vi "example_send_receive_raw.vi"() -> ()   [LabVIEW 2012]
doc: "EXAMPLE: Send / Receive Raw Data\n\nThis example VI allows the user to send and receive raw commands as outlined in the ASCII Language Specification of the USB Communication documentation. Simply key in the \"raw\" command string in the \"command (raw)\" field and run the VI to see the response.\n\nProduced By:\n\nChristopher Lemieux\nKod Integrations, LLC\n4835 Marianne Drive\nMount Airy, MD 21771\nhttp://www.kodintegrations.com\nemail: clemieux@kodintegrations.com\nphone: (240) 687-1288"
panel:
  in  "command (raw)":string
  in  "device_index (def=0)":i32
  out "response (raw)":string
  out "error out":errorcluster
  in  "error in (no error)":errorcluster
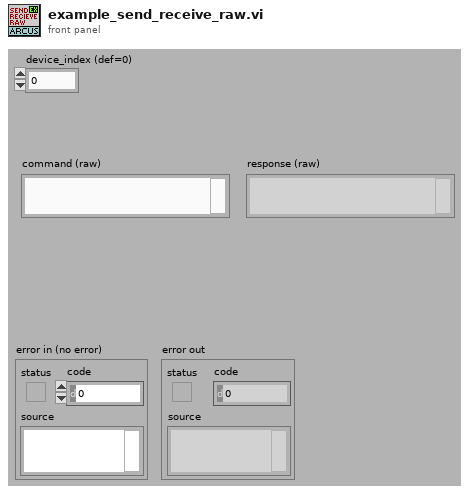
[diagram p1: front panel]
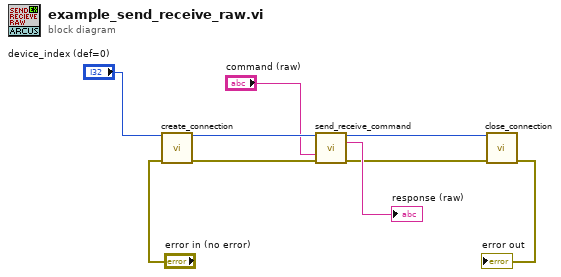
[diagram p0: block diagram]
diagram:
  n1 = call "create_connection.vi"("device_index (def=0)"="device_index (def=0)", "error in (no error)"="error in (no error)") -> ("reference"=w9:i32, "error out"=w8:errorcluster)  [unwired: 12 in]
  n2 = call "send_receive_command.vi"("reference (in)"=w9, "command (raw)"="command (raw)", "error in (no error)"=w8) -> ("reference (dup)"=w2:i32, "read_string"=→"response (raw)":string, "error out"=w3:errorcluster)  [unwired: 8 in, 2 out]
  n3 = call "close_connection.vi"("reference"=w2, "error in (no error)"=w3) -> ("error out"=→"error out":errorcluster)  [unwired: 13 in]
